vi "MCS_Homing.vi"(1 "error in (no error)":errorcluster, 2 "Direction":T1(ring), 3 "Channel Index In":u32, 4 "System Index In":u32) -> (0 "error out":errorcluster)   [LabVIEW 2010]
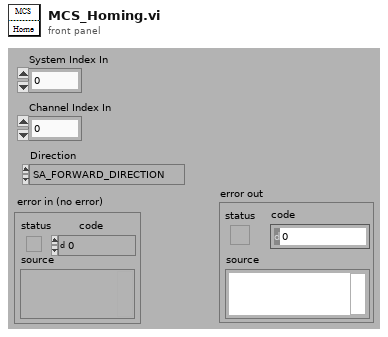
[diagram p1: front panel]
types:
  T1 = enum32{"SA_FORWARD_DIRECTION", "SA_BACKWARD_DIRECTION", "SA_FORWARD_BACKWARD_DIRECTION", "SA_BACKWARD_FORWARD_DIRECTION"}
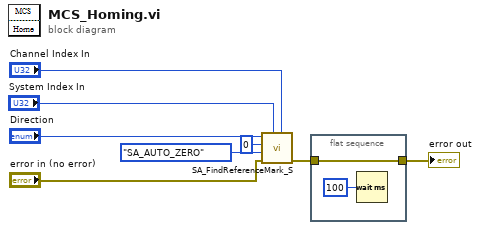
[diagram p0: block diagram]
diagram:
  n1 = call <vilib>:"SA_FindReferenceMark_S.vi"("channelIndex"="Channel Index In", "systemIndex"="System Index In", "error in (no error)"="error in (no error)", "autoZero"=enum32{"SA_NO_AUTO_ZERO", "SA_AUTO_ZERO"}."SA_AUTO_ZERO", "holdTime"=u32 0, "direction"="Direction") -> ("error out"=w2:errorcluster)  [unwired: 5 in]
  n2 = flat-sequence {
    tunnel: w2 -> [w9]
    tunnel: [w9] -> w1
    frame #0 {
      n3 = Wait (ms)(milliseconds to wait=u32 100) -> ()  [unwired: 1 out]
    }
  }
  "error out" <- w1
